vi "Add Tag to Experiment.vi"(8 "error in (no error)":errorcluster, 9 "tag":string, 10 "experiment id":u32, 11 "eLab in":refnum<class "PL eLabFTW Client.lvclass">) -> (0 "error out":errorcluster, 3 "eLab out":refnum<class "PL eLabFTW Client.lvclass">)   [LabVIEW 2015, in "PL eLabFTW Client.lvclass"]
doc: "Adds tag to the experiment."
uses:
  PL eLabFTW Client.lvclass
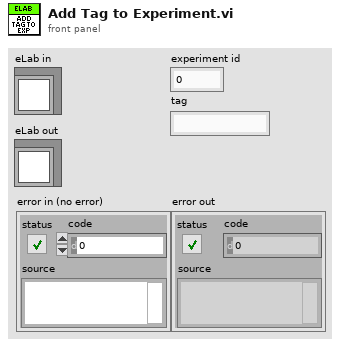
[diagram p1: front panel]
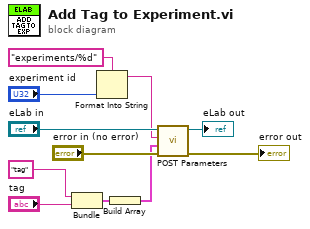
[diagram p0: block diagram]
diagram:
  n1 = Bundle("format string"="tag", "tag"="tag") -> (w4:cluster{"format string":string, "tag":string})  [unwired: 1 in]
  n2 = Format Into String(format string="experiments/%d", "experiment id") -> (resulting string=w5:string)  [unwired: 2 in, 1 out]
  n3 = Build Array(w4) -> (w1:cluster{"format string":string, "tag":string}[])
  n4 = call "POST Parameters.vi"("error in (no error)"="error in (no error)", "parameters"=w1, "relative URL"=w5, "eLab in"="eLab in") -> ("error out"=→"error out":errorcluster, "eLab out"=→"eLab out":refnum<class "PL eLabFTW Client.lvclass">)  [unwired: 5 in, 1 out]
